vi "non recursive akhil2.vi"() -> ()   [LabVIEW 2014]
uses:
  <vilib>/LabVIEW Targets/FPGA/cRIO/shared/nicrio_ModuleControls/nicrio_cRIO-9467_Altitude.ctl
  <vilib>/LabVIEW Targets/FPGA/cRIO/shared/nicrio_ModuleControls/nicrio_cRIO-9467_Longitude.ctl
  <vilib>/LabVIEW Targets/FPGA/cRIO/shared/nicrio_ModuleControls/nicrio_cRIO-9467_Latitude.ctl
  <vilib>/LabVIEW Targets/FPGA/cRIO/shared/nicrio_ModuleControls/nicrio_cRIO-9225_DataRatesRing.ctl
  <vilib>/LabVIEW Targets/FPGA/cRIO/shared/nicrio_ModuleControls/nicrio_cRIO-9227_DataRatesRing.ctl
  <vilib>/Platform/TimedLoop/XDataNode/timing_clust.ctl
  <vilib>/Platform/TimedLoop/XDataNode/nitl_modes.ctl
  <vilib>/Platform/TimedLoop/XDataNode/wakeup.ctl
  <vilib>/rvi/FXPMathLib/FxpSinAndCos/subVIs/nifxpmath_SinAndCos_SimConfig.ctl
  <vilib>/rvi/FXPMathLib/FxpRectToPolar/subVIs/nifxpmath_RectToPolar_SimConfig.ctl
  <vilib>/rvi/Emulation/niFpgaGetClockAttributes.vi
  <vilib>/rvi/Emulation/niFpgaSctlEmulationGetInTimedLoop.vi
  <vilib>/rvi/Emulation/niFpgaEmulationReportErrorSimple.vi
  <vilib>/rvi/eio/common/nirviEmuTemplateMethod_errors.vi
  <vilib>/rvi/eio/common/nirviEmuTemplatePropertyGet_noerrors.vi
  <vilib>/rvi/Emulation/niFpgaCriticalErrorInLSC.vi
  <vilib>/rvi/Memory/Memory_Emulation/nirvimemoryFastEmulation.vi
  <vilib>/rvi/Memory/Memory_Emulation/nirvimemoryEmulation.vi
  <vilib>/rvi/Emulation/niFpgaEmulationIsFPGAContextNoSignature.vi
  <vilib>/rvi/DataTransferAndStorage/Container/Common/niFpgaContainerGetUniqueNameForEmu.vi
  <vilib>/rvi/Emulation/niFpgaProcessEmulError.vi
  <vilib>/rvi/errors/nirviReportUnexpectedCaseInternalError (U32).vi
  <vilib>/rvi/FXPMathLib/FxpSinAndCos/simVIs/DllFxpSinAndCosTemp_sub.vi
  <vilib>/rvi/FXPMathLib/FxpRectToPolar/simVIs/DllFxpRectToPolarTemp_sub.vi
  <vilib>/rvi/DataTransferAndStorage/Container/Common/niFpgaContainerSetEmuInfo.vi
  <vilib>/rvi/eio/common/nirviEmuReportErrorAndStop.vi
  <vilib>/rvi/eio/common/nirviEmuTemplatePropertySet_noerrors.vi
  <vilib>/rvi/eio/common/nirviEmuTemplatePropertyGet_errors.vi
  <vilib>/eio/EIOMethodNode/EIOMethodNode.xnode
  <vilib>/eio/EIOPropertyNode/EIOPropertyNode.xnode
  <vilib>/eio/EIONode/EIONode.xnode
  <vilib>/Platform/TimedLoop/XDataNode/XDataNode.xnode
  <vilib>/rvi/DataTransferAndStorage/Container/XNode/niFpgaContainer.xnode
  <vilib>/rvi/FXPMathLib/FxpMul/XNode/nifxpmath_Multiplier.xnode
  <vilib>/rvi/FXPMathLib/FxpSinAndCos/XNode/nifxpmath_SinAndCos.xnode
  <vilib>/rvi/FXPMathLib/FxpAdd/XNode/nifxpmath_Add.xnode
  <vilib>/rvi/FXPMathLib/FxpRectToPolar/XNode/nifxpmath_RectToPolar.xnode
  <vilib>/rvi/LocalResourceManager/LocalResourceManager.xnode
  <vilib>/rvi/FXPMathLib/sim/FxpSim.dll
  <vilib>/Platform/TimedLoop/XDataNode/XDNodeRunTimeDep.lvlib
  <vilib>/rvi/eio/common/nirviEmuTemplatePropertySet_errors.vi
  fpga timekeeper/FPGA Timekeeper.lvlib
panel:
  out "Firmware Version":u32 format="%.0x"
  out "Vendor ID":u16 format="%.0x"
  out "Module ID":u16 format="%.0x"
  out "Serial Number":u32 format="%.0x"
  out "FPGA Error Out":errorcluster
  in  "stop 2":bool
  out "PPS Timestamp (TAI)":u64
  out "UTC Offset":i8
  out "UTC Offset Valid":bool
  out "GPS Status":T1(ring)
  out "Antenna Status":T2(ring)
  out "Leap Second Direction":enum8{"Add", "Delete"}(ring)
  out "Leap Second Pending":bool
  out "Leap Second Occurred":bool
  out "Satellites Available":u8
  out "Self-Survey Complete":bool
  out "Latitude (°)":T3 format="%.6f"
  out "Longitude (°)":T4 format="%.6g"
  out "Altitude (m)":T5 format="%.2f"
  out "Timed Out":bool
  out "Iterations":i32
  out "FPGA Timekeeper time (ns)":u64
  out "GPS status":T1(ring)
  out "FPGA Timekeeper locked":bool
  out "offset from time reference":i32
  out "antenna status":T2(ring)
  out "satellites available":u8
  out "UTC offset":i8
  out "UTC offset valid":bool
  out "rate of chage of frequency":fxp<+/-,26,12>
  out "phase current":fxp<+/-,26,12>
  out "phase voltage":fxp<+/-,26,12>
  out "current frequency":fxp<+/-,50,19>
  out "voltage frequency":fxp<+/-,50,19>
  out "sdft magnitude":fxp<+/-,25,11>[](array[numeric])
  out "sdft phase":fxp<+/-,25,11>[](array[numeric])
  out "y phase voltage":T6(array[cluster])
  out "y phase current":T6(array[cluster])
  out "r phase current":T6(array[cluster])
  out "r phase voltage":T6(array[cluster])
  out "b phase current":T6(array[cluster])
  out "b phase voltage":T6(array[cluster])
  out "Array":T7(array[cluster])
  out "theta":fxp<+/-,22,10>[](array[numeric])
  out "r":fxp<+,60,17>[](array[numeric])
  in  "stop":bool
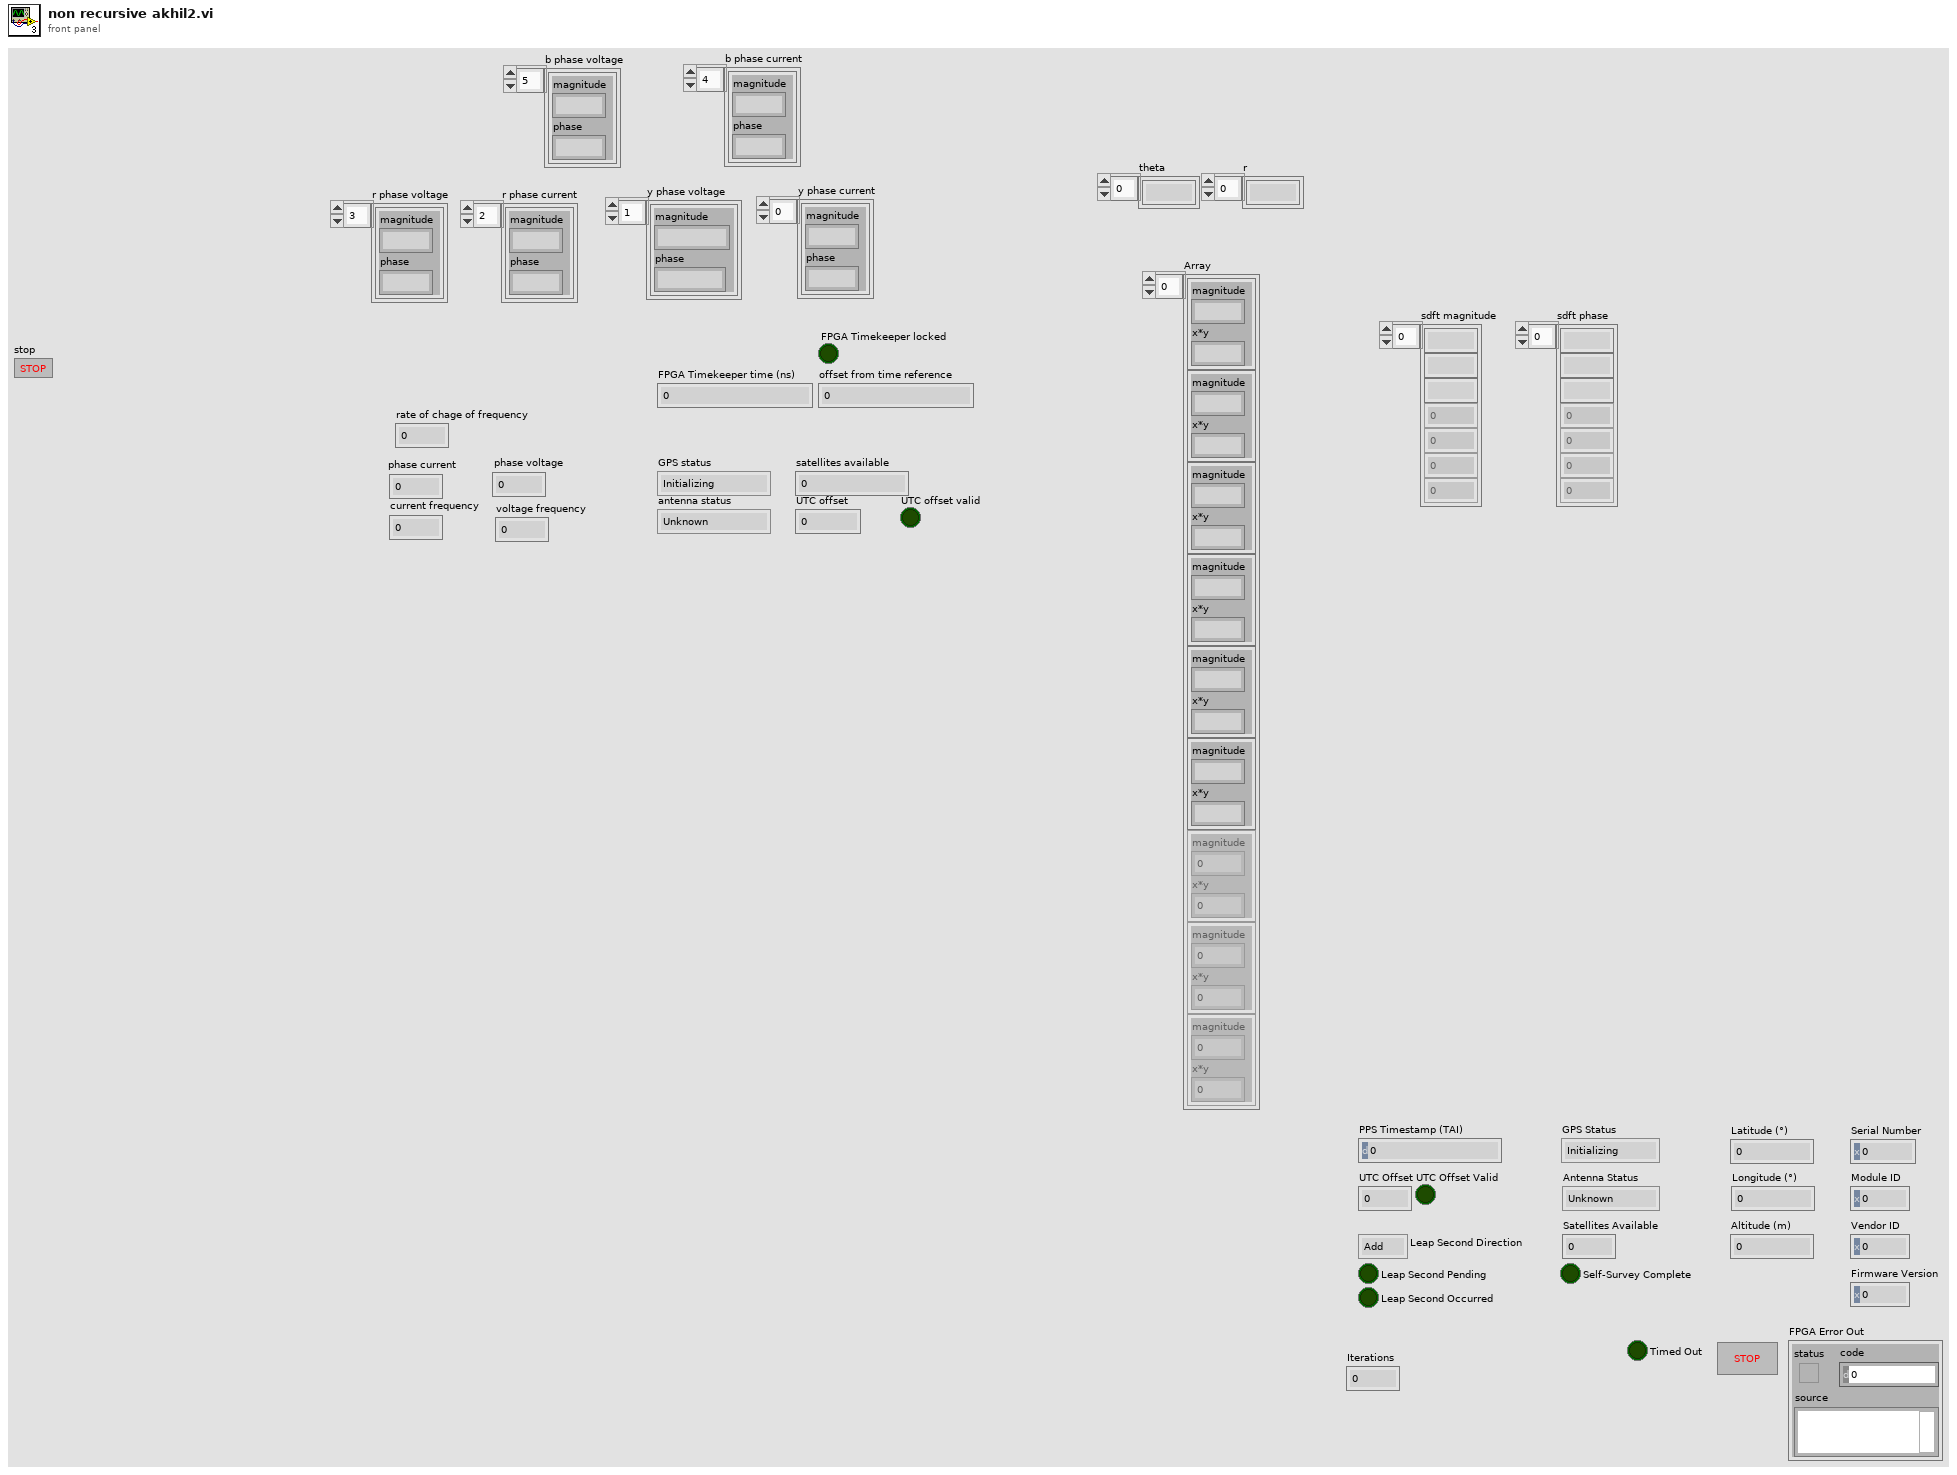
[diagram p1: front panel]
types:
  T1 = enum8{"Initializing", "Normal", "Unable to get fix"}
  T2 = enum8{"Unknown", "Normal", "Absent", "Overcurrent"}
  T3 = typedef "nicrio_cRIO-9467_Latitude.ctl" = fxp<+/-,28,8>
  T4 = typedef "nicrio_cRIO-9467_Longitude.ctl" = fxp<+/-,29,9>
  T5 = typedef "nicrio_cRIO-9467_Altitude.ctl" = fxp<+/-,24,17>
  T6 = cluster{"magnitude":fxp<+,60,17>, "phase":fxp<+/-,22,10>}[]
  T7 = cluster{"magnitude":fxp<+,60,17>, "x*y":fxp<+/-,22,10>}[]
  T8 = typedef "nicrio_cRIO-9227_DataRatesRing.ctl" = u8
  T9 = typedef "nicrio_cRIO-9225_DataRatesRing.ctl" = u8
  T10 = typedef "XDNodeRunTimeDep.lvlib/timing_clust.ctl" = cluster{"Expected End [f-1]":u64, "Actual End [f-1]":u64, "Finished Late? [f-1]":bool, "Expected End [i-1]":u64, "Actual End [i-1]":u64, "Finished Late? [i-1]":bool, "Expected Start [i]":u64, "Actual Start [i]":u64, "Expected Start [f]":u64, "Actual Start [f]":u64, "Source Name":string, "Structure Name":string, "Period":i64, "Deadline":i64, "Offset":i64, "Start":i64, "Priority":i32, "Timeout":i32, "Mode":T11, "Wakeup Reason":T12, "Error":errorcluster, "Source Type":string, "Secondary Source Type":string, "Global End Time":u64, "Global Start Time":u64, "Frame Duration":u64, "Iteration Duration":u64, "Assigned CPU":i32, "I/O Scan Engine Mode":u32}
  T11 = typedef "XDNodeRunTimeDep.lvlib/nitl_modes.ctl" = enum32{"No Change", "Process missed periods, maintain original phase", "Discard missed periods, maintain original phase", "Process missed periods, ignore original phase", "Discard missed periods, ignore original phase"}
  T12 = typedef "XDNodeRunTimeDep.lvlib/wakeup.ctl" = enum32{"Normal", "Aborted", "Asynchronous wakeup", "Timing source error", "Timed loop error", "Timeout"}
  T13 = cluster{"magnitude":fxp<+,60,17>, "x*y":fxp<+/-,22,10>}
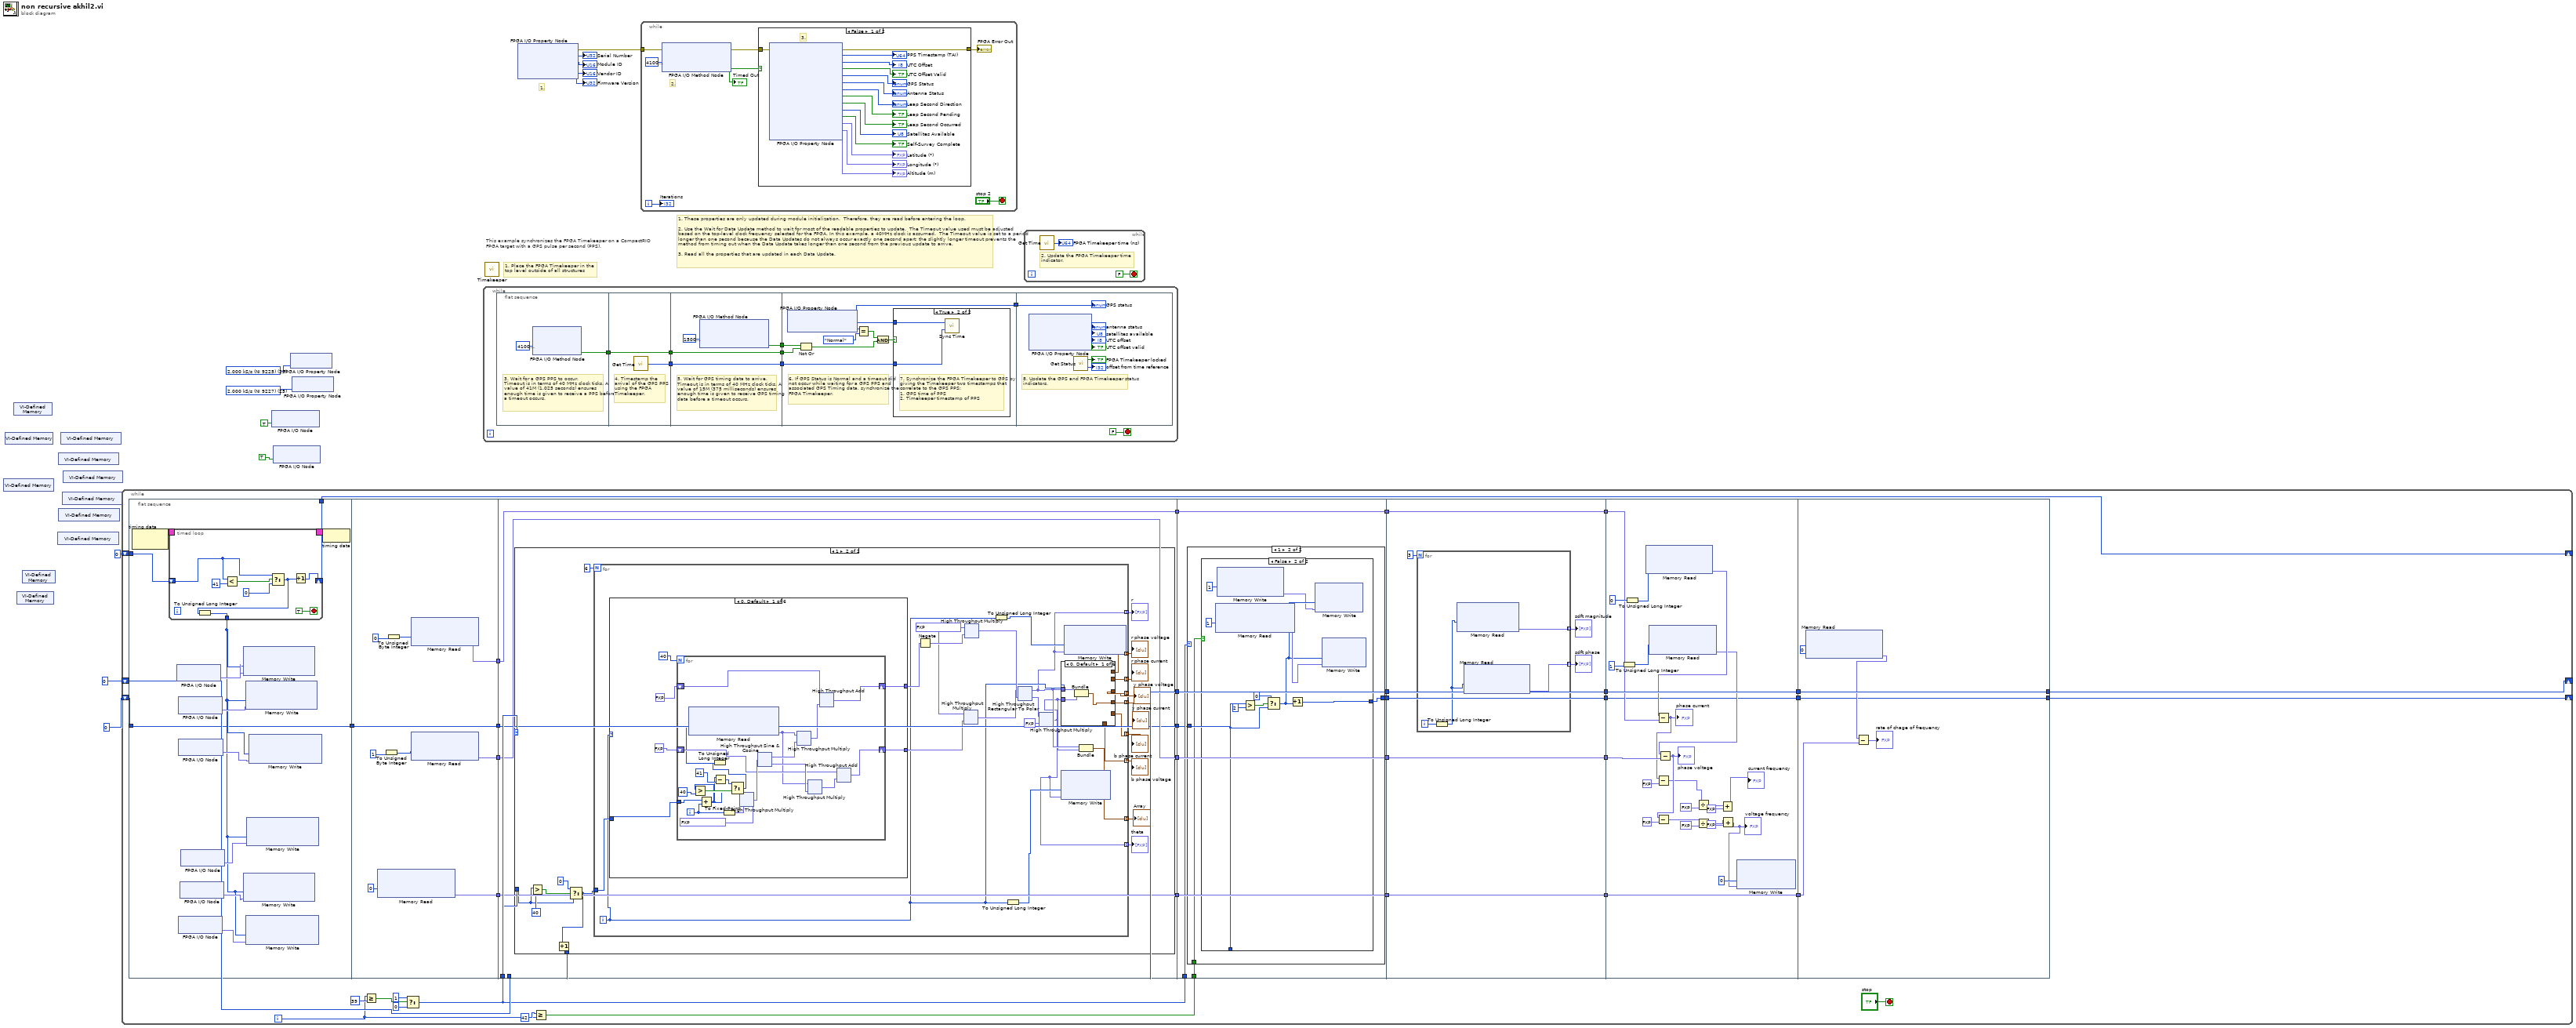
[diagram p0: block diagram]
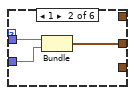
[diagram p5: hidden frame]
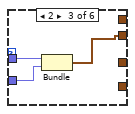
[diagram p6: hidden frame]
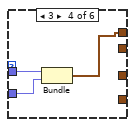
[diagram p7: hidden frame]
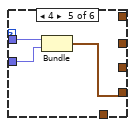
[diagram p8: hidden frame]
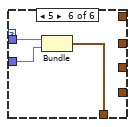
[diagram p9: hidden frame]
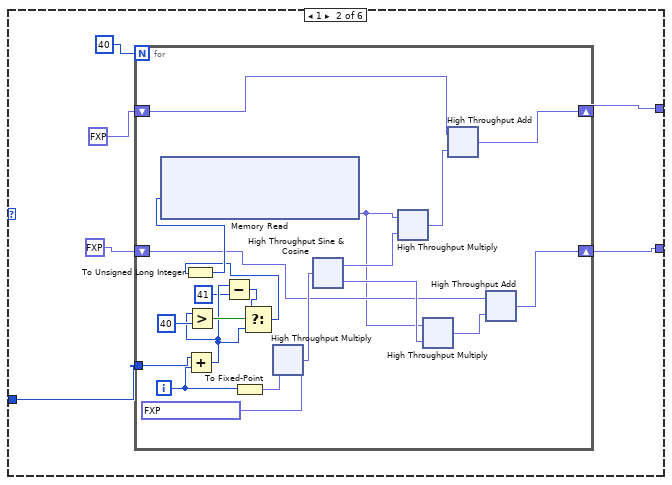
[diagram p10: hidden frame]
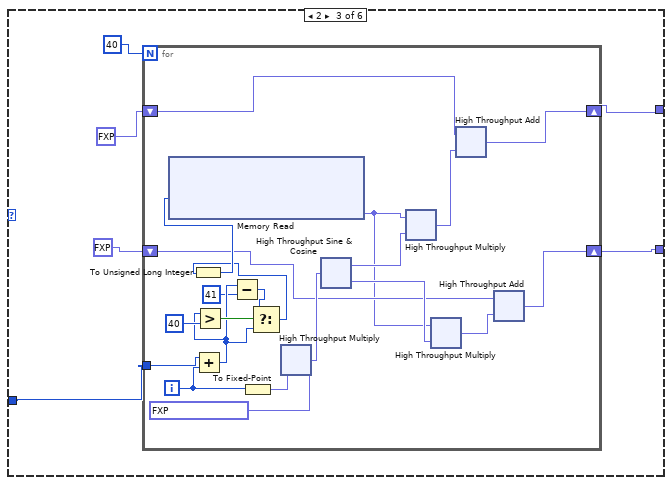
[diagram p11: hidden frame]
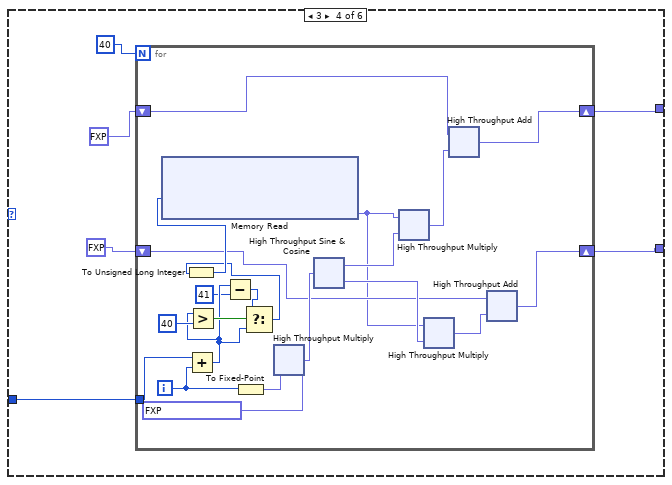
[diagram p12: hidden frame]
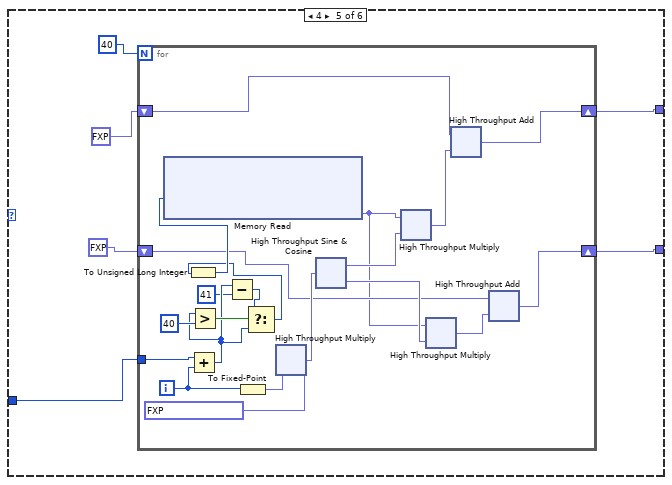
[diagram p13: hidden frame]
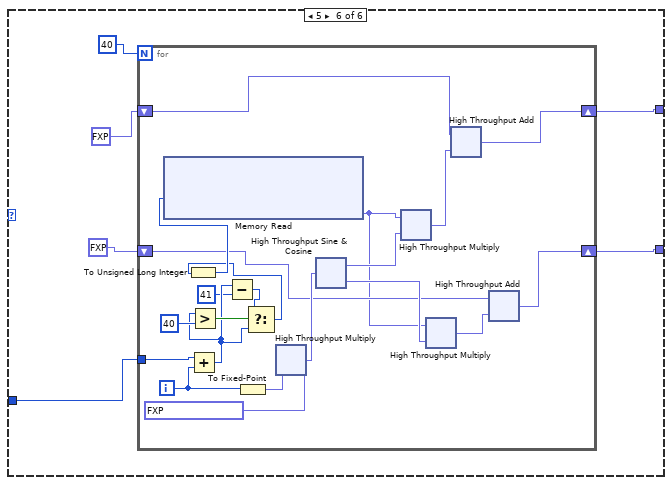
[diagram p14: hidden frame]
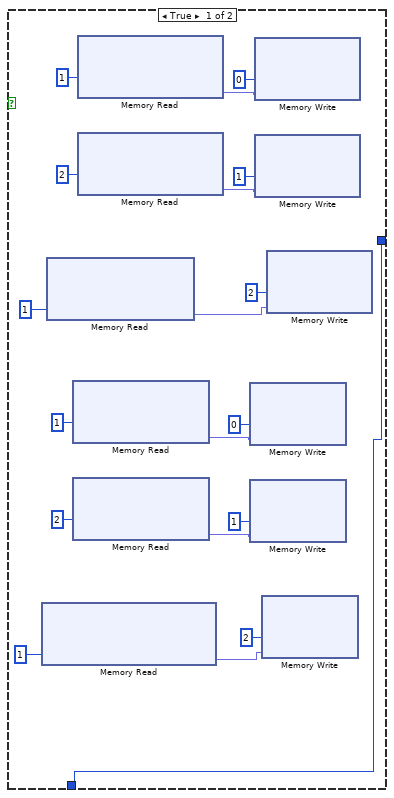
[diagram p16: hidden frame]
diagram:
  w11 = T8 25 items=["50.000 kS/s (NI 9227)"=1, "25.000 kS/s (NI 9227)"=2, "16.667 kS/s (NI 9227)"=3, "12.500 kS/s (NI 9227)"=4, "10.000 kS/s (NI 9227)"=5, "8.333 kS/s (NI 9227)"=6, "7.143 kS/s (NI 9227)"=7, "6.250 kS/s (NI 9227)"=8, "5.556 kS/s (NI 9227)"=9, "5.000 kS/s (NI 9227)"=10, "4.545 kS/s (NI 9227)"=11, "4.167 kS/s (NI 9227)"=12, "3.846 kS/s (NI 9227)"=13, "3.571 kS/s (NI 9227)"=14, "3.333 kS/s (NI 9227)"=15, "3.125 kS/s (NI 9227)"=16, "2.941 kS/s (NI 9227)"=17, "2.778 kS/s (NI 9227)"=18, "2.632 kS/s (NI 9227)"=19, "2.500 kS/s (NI 9227)"=20, "2.381 kS/s (NI 9227)"=21, "2.273 kS/s (NI 9227)"=22, "2.174 kS/s (NI 9227)"=23, "2.083 kS/s (NI 9227)"=24, "2.000 kS/s (NI 9227)"=25, "1.923 kS/s (NI 9227)"=26, "1.852 kS/s (NI 9227)"=27, "1.786 kS/s (NI 9227)"=28, "1.724 kS/s (NI 9227)"=29, "1.667 kS/s (NI 9227)"=30, "1.613 kS/s (NI 9227)"=31] ("Data Rate")
  w8 = T9 25 items=["50.000 kS/s (NI 9225)"=1, "25.000 kS/s (NI 9225)"=2, "16.667 kS/s (NI 9225)"=3, "12.500 kS/s (NI 9225)"=4, "10.000 kS/s (NI 9225)"=5, "8.333 kS/s (NI 9225)"=6, "7.143 kS/s (NI 9225)"=7, "6.250 kS/s (NI 9225)"=8, "5.556 kS/s (NI 9225)"=9, "5.000 kS/s (NI 9225)"=10, "4.545 kS/s (NI 9225)"=11, "4.167 kS/s (NI 9225)"=12, "3.846 kS/s (NI 9225)"=13, "3.571 kS/s (NI 9225)"=14, "3.333 kS/s (NI 9225)"=15, "3.125 kS/s (NI 9225)"=16, "2.941 kS/s (NI 9225)"=17, "2.778 kS/s (NI 9225)"=18, "2.632 kS/s (NI 9225)"=19, "2.500 kS/s (NI 9225)"=20, "2.381 kS/s (NI 9225)"=21, "2.273 kS/s (NI 9225)"=22, "2.174 kS/s (NI 9225)"=23, "2.083 kS/s (NI 9225)"=24, "2.000 kS/s (NI 9225)"=25, "1.923 kS/s (NI 9225)"=26, "1.852 kS/s (NI 9225)"=27, "1.786 kS/s (NI 9225)"=28, "1.724 kS/s (NI 9225)"=29, "1.667 kS/s (NI 9225)"=30, "1.613 kS/s (NI 9225)"=31] ("Data Rate")
  # "1."
  # "1. These properties are only updated during module initialization.  Therefore, they are read before entering the loop.\n\n2. Use the Wait for Data Update method to wait for most of the readable properties to update.  The Timeout value used must be adjusted based on the top-level clock frequency selected for the FPGA. In this example, a 40MHz clock is assumed.  The Timeout value is set to a period longer than one second because the Data Updates do not always occur exactly one second apart; the slightly longer timeout prevents the method from timing out when the Data Update takes longer than one second from the previous update to arrive. \n\n3. Read all the properties that are updated in each Data Update."
  # "This example synchronizes the FPGA Timekeeper on a CompactRIO FPGA target with a GPS pulse per second (PPS)."
  # "1. Place the FPGA Timekeeper in the\ntop level outside of all structures"
  n1 = xnode "VI-Defined Memory"() -> ()  [unwired: 1 out]
  n2 = xnode "VI-Defined Memory"() -> ()  [unwired: 1 out]
  n3 = xnode "VI-Defined Memory"() -> ()  [unwired: 1 out]
  n4 = xnode "VI-Defined Memory"() -> ()  [unwired: 1 out]
  n5 = xnode "VI-Defined Memory"() -> ()  [unwired: 1 out]
  n6 = xnode "VI-Defined Memory"() -> ()  [unwired: 1 out]
  n7 = xnode "VI-Defined Memory"() -> ()  [unwired: 1 out]
  n8 = xnode "VI-Defined Memory"() -> ()  [unwired: 1 out]
  n9 = xnode "VI-Defined Memory"() -> ()  [unwired: 1 out]
  n10 = xnode "VI-Defined Memory"() -> ()  [unwired: 1 out]
  n11 = xnode "VI-Defined Memory"() -> ()  [unwired: 1 out]
  n12 = while {
    shift-right: [w48] -> _
    shift-left: i16 0 -> [w49]
    shift-right: [w42] -> _
    shift-left: u32 0 ("t") -> [w43]
    shift-right: [w21] -> _
    shift-left: u32 0 ("t") -> [w33]
    i -> [w20]
    stop <- "stop" stop-if-true
    n13 = flat-sequence {
      tunnel: w49 -> [w61]
      tunnel: [w60] -> w48
      tunnel: [w51] -> w34
      tunnel: w33 -> [w51]
      tunnel: [w79] -> w41
      tunnel: [w78] -> w40
      tunnel: [w76] -> w37
      tunnel: [w75] -> w35
      tunnel: w34 -> [w75]
      tunnel: w36 -> [w90]
      tunnel: w43 -> [w89]
      tunnel: [w88] -> w17
      tunnel: w41 -> [w87]
      tunnel: [w87] -> w16
      tunnel: [w86] -> w15
      tunnel: w40 -> [w86]
      tunnel: [w85] -> w14
      tunnel: w37 -> [w85]
      tunnel: [w84] -> w13
      tunnel: w35 -> [w84]
      tunnel: w17 -> [w533]
      tunnel: [w533] -> w31
      tunnel: w16 -> [w532]
      tunnel: [w532] -> w29
      tunnel: w15 -> [w531]
      tunnel: [w531] -> w27
      tunnel: w14 -> [w530]
      tunnel: [w530] -> w25
      tunnel: w36 -> [w529]
      tunnel: w13 -> [w528]
      tunnel: [w527] -> w23
      tunnel: w18 -> [w526]
      tunnel: w31 -> [w574]
      tunnel: [w574] -> w30
      tunnel: w29 -> [w573]
      tunnel: [w573] -> w28
      tunnel: w27 -> [w572]
      tunnel: [w572] -> w26
      tunnel: w25 -> [w571]
      tunnel: [w571] -> w24
      tunnel: w23 -> [w570]
      tunnel: [w570] -> w22
      tunnel: w30 -> [w604]
      tunnel: w28 -> [w599]
      tunnel: w26 -> [w598]
      tunnel: [w604] -> w39
      tunnel: [w580] -> w38
      tunnel: w24 -> [w580]
      tunnel: [w579] -> w32
      tunnel: w22 -> [w579]
      tunnel: [w610] -> w42
      tunnel: w39 -> [w610]
      tunnel: w38 -> [w608]
      tunnel: [w605] -> w21
      tunnel: w32 -> [w605]
      frame #0 {
        n14 = node-c288() -> (w53:T10)  [unwired: 1 in]
        n15 = timed-loop {
          timing: w53 -> [_]
          timing-out: [_] -> w52
          tunnel: [w64] -> w54
          shift-right: [w65] -> w60
          shift-left: w61 -> [w66]
          stop <- TRUE stop-if-true
          n16 = Less?(x=w66, y=i16 41) -> (x < y?=w69:bool)
          n17 = Select(t=w66, s=w69, f=i16 0) -> (s? t:f=w67:i16)
          n18 = To Unsigned Long Integer(number=w67) -> (unsigned 32bit integer=w64:u32)
          n19 = Increment(x=w67) -> (x+1=w65:i16)
        }
        n20 = xnode "FPGA I/O Node"() -> ("Mod2/AI1"=w59:fxp<+/-,24,5>)  [unwired: 1 in, 1 out]
        n21 = xnode "FPGA I/O Node"() -> ("Mod2/AI0"=w56:fxp<+/-,24,5>)  [unwired: 1 in, 1 out]
        n22 = xnode "FPGA I/O Node"() -> ("Mod1/AI2"=w57:fxp<+/-,24,10>)  [unwired: 1 in, 1 out]
        n23 = xnode "FPGA I/O Node"() -> ("Mod2/AI2"=w55:fxp<+/-,24,5>)  [unwired: 1 in, 1 out]
        n24 = xnode "FPGA I/O Node"() -> ("Mod1/AI0"=w58:fxp<+/-,24,10>)  [unwired: 1 in, 1 out]
        n25 = xnode "FPGA I/O Node"() -> ("Mod1/AI1"=w62:fxp<+/-,24,10>)  [unwired: 1 in, 1 out]
        n26 = xnode ("Memory Write")("Address"=w54, "Data"=w59) -> ()  [unwired: 1 in, 1 out]
        n27 = xnode ("Memory Write")("Address"=w54, "Data"=w58) -> ()  [unwired: 1 in, 1 out]
        n28 = xnode ("Memory Write")("Address"=w54, "Data"=w56) -> ()  [unwired: 1 in, 1 out]
        n29 = xnode ("Memory Write")("Address"=w54, "Data"=w57) -> ()  [unwired: 1 in, 1 out]
        n30 = xnode ("Memory Write")("Address"=w54, "Data"=w62) -> ()  [unwired: 1 in, 1 out]
        n31 = xnode ("Memory Write")("Address"=w54, "Data"=w55) -> ()  [unwired: 1 in, 1 out]
        n32 = node-c288(w52) -> ()
      }
      frame #1 {
        n33 = xnode ("Memory Read")("Address"=u32 0) -> ("Data"=w76:fxp<+/-,25,11>)  [unwired: 1 in, 1 out]
        n34 = To Unsigned Byte Integer(number=i16 1) -> (unsigned 8bit integer=w80:u8)
        n35 = To Unsigned Byte Integer(number=i16 0) -> (unsigned 8bit integer=w82:u8)
        n36 = xnode ("Memory Read")("Address"=w82) -> ("Data"=w79:fxp<+/-,25,11>)  [unwired: 1 in, 1 out]
        n37 = xnode ("Memory Read")("Address"=w80) -> ("Data"=w78:fxp<+/-,25,11>)  [unwired: 1 in, 1 out]
      }
      frame #2 {
        n38 = case shown="1" w90 {
          tunnel: w89 -> [w91 w102]
          tunnel: [w91 w105] -> w88
          frame 0, Default {
          }
          frame 1 {
            n39 = Greater?(x=w102, y=u32 40) -> (0:w103:bool)
            n40 = Select(t=u32 0, s=w103, f=w102) -> (s? t:f=w100:u32)
            n41 = Increment(x=w100) -> (x+1=w105:u32)
            n42 = for {
              N: 6 -> [_]
              tunnel: [w121] -> w106 mode=indexing
              tunnel: w100 -> [w120]
              tunnel: [w116] -> w99 mode=indexing
              tunnel: [w115] -> w98 mode=indexing
              tunnel: [w114] -> w97 mode=indexing
              tunnel: [w113] -> w96 mode=indexing
              tunnel: [w112] -> w95 mode=indexing
              tunnel: [w110] -> w94 mode=indexing
              tunnel: [w108] -> w93 mode=indexing
              tunnel: [w109] -> w92 mode=indexing
              i -> [w117]
              w127 = fxp<+/-,16,1> 0.03533935546875 ("x")
              n43 = case shown="0, Default" w117 {
                tunnel: [w185 w241 w298 w355 w412 w469] -> w122
                tunnel: w120 -> [w184 w243 w300 w357 w414 w471]
                tunnel: [w186 w242 w299 w356 w413 w470] -> w119
                frame 0, Default {
                  n44 = for {
                    N: 40 ("Numeric") -> [_]
                    shift-right: [w203] -> w185
                    shift-left: fxp<+,1,1> 0.0 ("x+y") -> [w202]
                    shift-right: [w206] -> w186
                    shift-left: fxp<+,1,1> 0.0 -> [w201]
                    tunnel: w184 -> [w193]
                    i -> [w194]
                    n45 = Add(x=w193, y=w194) -> (x+y=w192:u32)
                    n46 = Greater?(x=w192, y=u32 40) -> (0:w197:bool)
                    n47 = Subtract(x=w192, y=u32 41) -> (x-y=w195:u32)
                    n48 = To Fixed-Point(number=w194) -> (fixed-point=w210:fxp<+/-,32,32>)  [unwired: 1 in]
                    n49 = Select(t=w195, s=w197, f=w192) -> (s? t:f=w191:u32)
                    n50 = To Unsigned Long Integer(number=w191) -> (unsigned 32bit integer=w190:u32)
                    n51 = xnode ("Memory Read")("Address"=w190) -> ("Data"=w199:fxp<+/-,25,11>)  [unwired: 1 in, 1 out]
                    n52 = xnode ("High Throughput Multiply")("x"=fxp<+/-,32,16> 0.04998779296875 ("number"), "y"=w210) -> ("x*y"=w209:fxp<+/-,64,48>)
                    n53 = xnode "High Throughput Sine & Cosine"("x (pi)"=w209) -> ("sin(x)"=w208:fxp<+/-,16,2>, "cos(x)"=w205:fxp<+/-,16,2>)
                    n54 = xnode ("High Throughput Multiply")("x"=w199, "y"=w208) -> ("x*y"=w207:fxp<+/-,41,13>)
                    n55 = xnode ("High Throughput Multiply")("x"=w199, "y"=w205) -> ("x*y"=w204:fxp<+/-,41,13>)
                    n56 = xnode ("High Throughput Add")("x"=w201, "y"=w207) -> ("x+y"=w206:fxp<+/-,42,14>)
                    n57 = xnode ("High Throughput Add")("x"=w202, "y"=w204) -> ("x+y"=w203:fxp<+/-,44,16>)
                  }
                }
                frame 1 {
                  n58 = for {
                    N: 40 ("Numeric") -> [_]
                    shift-right: [w259] -> w241
                    shift-left: fxp<+,1,1> 0.0 ("x+y") -> [w258]
                    shift-right: [w262] -> w242
                    shift-left: fxp<+,1,1> 0.0 -> [w257]
                    tunnel: w243 -> [w254]
                    i -> [w253]
                    n59 = Add(x=w254, y=w253) -> (x+y=w249:u32)
                    n60 = Greater?(x=w249, y=u32 40) -> (0:w251:bool)
                    n61 = Subtract(x=w249, y=u32 41) -> (x-y=w247:u32)
                    n62 = To Fixed-Point(number=w253) -> (fixed-point=w266:fxp<+/-,32,32>)  [unwired: 1 in]
                    n63 = Select(t=w247, s=w251, f=w249) -> (s? t:f=w250:u32)
                    n64 = To Unsigned Long Integer(number=w250) -> (unsigned 32bit integer=w267:u32)
                    n65 = xnode ("Memory Read")("Address"=w267) -> ("Data"=w255:fxp<+/-,25,11>)  [unwired: 1 in, 1 out]
                    n66 = xnode ("High Throughput Multiply")("x"=fxp<+/-,32,16> 0.04998779296875 ("number"), "y"=w266) -> ("x*y"=w265:fxp<+/-,64,48>)
                    n67 = xnode "High Throughput Sine & Cosine"("x (pi)"=w265) -> ("sin(x)"=w264:fxp<+/-,16,2>, "cos(x)"=w261:fxp<+/-,16,2>)
                    n68 = xnode ("High Throughput Multiply")("x"=w255, "y"=w264) -> ("x*y"=w263:fxp<+/-,41,13>)
                    n69 = xnode ("High Throughput Multiply")("x"=w255, "y"=w261) -> ("x*y"=w260:fxp<+/-,41,13>)
                    n70 = xnode ("High Throughput Add")("x"=w257, "y"=w263) -> ("x+y"=w262:fxp<+/-,42,14>)
                    n71 = xnode ("High Throughput Add")("x"=w258, "y"=w260) -> ("x+y"=w259:fxp<+/-,44,16>)
                  }
                }
                frame 2 {
                  n72 = for {
                    N: 40 ("Numeric") -> [_]
                    shift-right: [w316] -> w298
                    shift-left: fxp<+,1,1> 0.0 ("x+y") -> [w315]
                    shift-right: [w319] -> w299
                    shift-left: fxp<+,1,1> 0.0 -> [w314]
                    tunnel: w300 -> [w311]
                    i -> [w310]
                    n73 = Add(x=w311, y=w310) -> (x+y=w306:u32)
                    n74 = Greater?(x=w306, y=u32 40) -> (0:w308:bool)
                    n75 = Subtract(x=w306, y=u32 41) -> (x-y=w304:u32)
                    n76 = To Fixed-Point(number=w310) -> (fixed-point=w323:fxp<+/-,32,32>)  [unwired: 1 in]
                    n77 = Select(t=w304, s=w308, f=w306) -> (s? t:f=w307:u32)
                    n78 = To Unsigned Long Integer(number=w307) -> (unsigned 32bit integer=w324:u32)
                    n79 = xnode ("Memory Read")("Address"=w324) -> ("Data"=w312:fxp<+/-,25,11>)  [unwired: 1 in, 1 out]
                    n80 = xnode ("High Throughput Multiply")("x"=fxp<+/-,32,16> 0.04998779296875 ("number"), "y"=w323) -> ("x*y"=w322:fxp<+/-,64,48>)
                    n81 = xnode "High Throughput Sine & Cosine"("x (pi)"=w322) -> ("sin(x)"=w321:fxp<+/-,16,2>, "cos(x)"=w318:fxp<+/-,16,2>)
                    n82 = xnode ("High Throughput Multiply")("x"=w312, "y"=w321) -> ("x*y"=w320:fxp<+/-,41,13>)
                    n83 = xnode ("High Throughput Multiply")("x"=w312, "y"=w318) -> ("x*y"=w317:fxp<+/-,41,13>)
                    n84 = xnode ("High Throughput Add")("x"=w314, "y"=w320) -> ("x+y"=w319:fxp<+/-,42,14>)
                    n85 = xnode ("High Throughput Add")("x"=w315, "y"=w317) -> ("x+y"=w316:fxp<+/-,44,16>)
                  }
                }
                frame 3 {
                  n86 = for {
                    N: 40 ("Numeric") -> [_]
                    shift-right: [w373] -> w355
                    shift-left: fxp<+,1,1> 0.0 ("x+y") -> [w372]
                    shift-right: [w376] -> w356
                    shift-left: fxp<+,1,1> 0.0 -> [w371]
                    tunnel: w357 -> [w361]
                    i -> [w368]
                    n87 = Add(x=w361, y=w368) -> (x+y=w364:u32)
                    n88 = Greater?(x=w364, y=u32 40) -> (0:w366:bool)
                    n89 = Subtract(x=w364, y=u32 41) -> (x-y=w362:u32)
                    n90 = To Fixed-Point(number=w368) -> (fixed-point=w380:fxp<+/-,32,32>)  [unwired: 1 in]
                    n91 = Select(t=w362, s=w366, f=w364) -> (s? t:f=w365:u32)
                    n92 = To Unsigned Long Integer(number=w365) -> (unsigned 32bit integer=w381:u32)
                    n93 = xnode ("Memory Read")("Address"=w381) -> ("Data"=w369:fxp<+/-,25,11>)  [unwired: 1 in, 1 out]
                    n94 = xnode ("High Throughput Multiply")("x"=fxp<+/-,32,16> 0.04998779296875 ("number"), "y"=w380) -> ("x*y"=w379:fxp<+/-,64,48>)
                    n95 = xnode "High Throughput Sine & Cosine"("x (pi)"=w379) -> ("sin(x)"=w378:fxp<+/-,16,2>, "cos(x)"=w375:fxp<+/-,16,2>)
                    n96 = xnode ("High Throughput Multiply")("x"=w369, "y"=w378) -> ("x*y"=w377:fxp<+/-,41,13>)
                    n97 = xnode ("High Throughput Multiply")("x"=w369, "y"=w375) -> ("x*y"=w374:fxp<+/-,41,13>)
                    n98 = xnode ("High Throughput Add")("x"=w371, "y"=w377) -> ("x+y"=w376:fxp<+/-,42,14>)
                    n99 = xnode ("High Throughput Add")("x"=w372, "y"=w374) -> ("x+y"=w373:fxp<+/-,44,16>)
                  }
                }
                frame 4 {
                  n100 = for {
                    N: 40 ("Numeric") -> [_]
                    shift-right: [w430] -> w412
                    shift-left: fxp<+,1,1> 0.0 ("x+y") -> [w429]
                    shift-right: [w433] -> w413
                    shift-left: fxp<+,1,1> 0.0 -> [w428]
                    tunnel: w414 -> [w418]
                    i -> [w425]
                    n101 = Add(x=w418, y=w425) -> (x+y=w421:u32)
                    n102 = Greater?(x=w421, y=u32 40) -> (0:w423:bool)
                    n103 = Subtract(x=w421, y=u32 41) -> (x-y=w419:u32)
                    n104 = To Fixed-Point(number=w425) -> (fixed-point=w437:fxp<+/-,32,32>)  [unwired: 1 in]
                    n105 = Select(t=w419, s=w423, f=w421) -> (s? t:f=w422:u32)
                    n106 = To Unsigned Long Integer(number=w422) -> (unsigned 32bit integer=w438:u32)
                    n107 = xnode ("Memory Read")("Address"=w438) -> ("Data"=w426:fxp<+/-,25,11>)  [unwired: 1 in, 1 out]
                    n108 = xnode ("High Throughput Multiply")("x"=fxp<+/-,32,16> 0.04998779296875 ("number"), "y"=w437) -> ("x*y"=w436:fxp<+/-,64,48>)
                    n109 = xnode "High Throughput Sine & Cosine"("x (pi)"=w436) -> ("sin(x)"=w435:fxp<+/-,16,2>, "cos(x)"=w432:fxp<+/-,16,2>)
                    n110 = xnode ("High Throughput Multiply")("x"=w426, "y"=w435) -> ("x*y"=w434:fxp<+/-,41,13>)
                    n111 = xnode ("High Throughput Multiply")("x"=w426, "y"=w432) -> ("x*y"=w431:fxp<+/-,41,13>)
                    n112 = xnode ("High Throughput Add")("x"=w428, "y"=w434) -> ("x+y"=w433:fxp<+/-,42,14>)
                    n113 = xnode ("High Throughput Add")("x"=w429, "y"=w431) -> ("x+y"=w430:fxp<+/-,44,16>)
                  }
                }
                frame 5 {
                  n114 = for {
                    N: 40 ("Numeric") -> [_]
                    shift-right: [w487] -> w469
                    shift-left: fxp<+,1,1> 0.0 ("x+y") -> [w486]
                    shift-right: [w490] -> w470
                    shift-left: fxp<+,1,1> 0.0 -> [w485]
                    tunnel: w471 -> [w475]
                    i -> [w482]
                    n115 = Add(x=w475, y=w482) -> (x+y=w478:u32)
                    n116 = Greater?(x=w478, y=u32 40) -> (0:w480:bool)
                    n117 = Subtract(x=w478, y=u32 41) -> (x-y=w476:u32)
                    n118 = To Fixed-Point(number=w482) -> (fixed-point=w494:fxp<+/-,32,32>)  [unwired: 1 in]
                    n119 = Select(t=w476, s=w480, f=w478) -> (s? t:f=w479:u32)
                    n120 = To Unsigned Long Integer(number=w479) -> (unsigned 32bit integer=w495:u32)
                    n121 = xnode ("Memory Read")("Address"=w495) -> ("Data"=w483:fxp<+/-,25,11>)  [unwired: 1 in, 1 out]
                    n122 = xnode ("High Throughput Multiply")("x"=fxp<+/-,32,16> 0.04998779296875 ("number"), "y"=w494) -> ("x*y"=w493:fxp<+/-,64,48>)
                    n123 = xnode "High Throughput Sine & Cosine"("x (pi)"=w493) -> ("sin(x)"=w492:fxp<+/-,16,2>, "cos(x)"=w489:fxp<+/-,16,2>)
                    n124 = xnode ("High Throughput Multiply")("x"=w483, "y"=w492) -> ("x*y"=w491:fxp<+/-,41,13>)
                    n125 = xnode ("High Throughput Multiply")("x"=w483, "y"=w489) -> ("x*y"=w488:fxp<+/-,41,13>)
                    n126 = xnode ("High Throughput Add")("x"=w485, "y"=w491) -> ("x+y"=w490:fxp<+/-,42,14>)
                    n127 = xnode ("High Throughput Add")("x"=w486, "y"=w488) -> ("x+y"=w487:fxp<+/-,44,16>)
                  }
                }
              }
              n128 = Negate(x=w119) -> (-x=w128:fxp<+/-,43,15>)
              n129 = xnode ("High Throughput Multiply")("x"=w127, "y"=w122) -> ("x*y"=w123:fxp<+/-,60,17>)
              n130 = xnode ("High Throughput Multiply")("x"=w127, "y"=w128) -> ("x*y"=w124:fxp<+/-,59,16>)
              n131 = To Unsigned Long Integer(number=w117) -> (unsigned 32bit integer=w111:u32)
              n132 = To Unsigned Long Integer(number=w117) -> (unsigned 32bit integer=w118:u32)
              n133 = xnode "High Throughput Rectangular To Polar"("x"=w123, "y"=w124) -> ("magnitude"=w109:fxp<+,60,17>, "phase (pi)"=w126:fxp<+/-,16,2>)
              n134 = xnode ("High Throughput Multiply")("x"=w126, "y"=fxp<+,6,8> 180.0) -> ("x*y"=w108:fxp<+/-,22,10>)
              n135 = case shown="0, Default" w117 {
                tunnel: [_ w134 _ _ _ _] -> w121
                tunnel: w108 -> [w131 w133 w137 w140 w143 w146]
                tunnel: w109 -> [w130 w132 w136 w139 w142 w145]
                tunnel: [w129 _ _ _ _ _] -> w116
                tunnel: [_ _ w135 _ _ _] -> w115
                tunnel: [_ _ _ w138 _ _] -> w114
                tunnel: [_ _ _ _ w141 _] -> w113
                tunnel: [_ _ _ _ _ w144] -> w112
                frame 0, Default {
                  n136 = Bundle("magnitude"=w130, "x*y"=w131) -> (w129:T13)  [unwired: 1 in]
                }
                frame 1 {
                  n137 = Bundle("magnitude"=w132, "x*y"=w133) -> (w134:T13)  [unwired: 1 in]
                }
                frame 2 {
                  n138 = Bundle("magnitude"=w136, "x*y"=w137) -> (w135:T13)  [unwired: 1 in]
                }
                frame 3 {
                  n139 = Bundle("magnitude"=w139, "x*y"=w140) -> (w138:T13)  [unwired: 1 in]
                }
                frame 4 {
                  n140 = Bundle("magnitude"=w142, "x*y"=w143) -> (w141:T13)  [unwired: 1 in]
                }
                frame 5 {
                  n141 = Bundle("magnitude"=w145, "x*y"=w146) -> (w144:T13)  [unwired: 1 in]
                }
              }
              n142 = xnode ("Memory Write")("Address"=w118, "Data"=w108) -> ()  [unwired: 1 in, 1 out]
              n143 = xnode ("Memory Write")("Address"=w111, "Data"=w109) -> ()  [unwired: 1 in, 1 out]
              n144 = Bundle("magnitude"=w109, "x*y"=w108) -> (w110:T13)  [unwired: 1 in]
            }
            "y phase voltage" <- w106
            "y phase current" <- w99
            "r phase current" <- w98
            "r phase voltage" <- w97
            "b phase current" <- w96
            "b phase voltage" <- w95
            "Array" <- w94
            "theta" <- w93
            "r" <- w92
          }
        }
      }
      frame #3 {
        n145 = case shown="1" w529 {
          tunnel: w528 -> [w534 w536]
          tunnel: [w534 w537] -> w527
          tunnel: w526 -> [_ w535]
          frame 0, Default {
          }
          frame 1 {
            n146 = case shown="False" w535 {
              tunnel: [w556 w564] -> w537
              tunnel: w536 -> [w556 w561]
              frame True {
                n147 = xnode ("Memory Read")("Address"=u32 1) -> ("Data"=w538:fxp<+/-,25,11>)  [unwired: 1 in, 1 out]
                n148 = xnode ("Memory Read")("Address"=u32 1) -> ("Data"=w547:fxp<+/-,25,11>)  [unwired: 1 in, 1 out]
                n149 = xnode ("Memory Read")("Address"=u32 1) -> ("Data"=w545:fxp<+/-,25,11>)  [unwired: 1 in, 1 out]
                n150 = xnode ("Memory Read")("Address"=u32 2) -> ("Data"=w542:fxp<+/-,25,11>)  [unwired: 1 in, 1 out]
                n151 = xnode ("Memory Read")("Address"=u32 1) -> ("Data"=w554:fxp<+/-,25,11>)  [unwired: 1 in, 1 out]
                n152 = xnode ("Memory Read")("Address"=u32 2) -> ("Data"=w551:fxp<+/-,25,11>)  [unwired: 1 in, 1 out]
                n153 = xnode ("Memory Write")("Address"=u32 0, "Data"=w545) -> ()  [unwired: 1 in, 1 out]
                n154 = xnode ("Memory Write")("Address"=u32 1, "Data"=w542) -> ()  [unwired: 1 in, 1 out]
                n155 = xnode ("Memory Write")("Address"=u32 0, "Data"=w554) -> ()  [unwired: 1 in, 1 out]
                n156 = xnode ("Memory Write")("Address"=u32 1, "Data"=w551) -> ()  [unwired: 1 in, 1 out]
                n157 = xnode ("Memory Write")("Address"=u32 2, "Data"=w538) -> ()  [unwired: 1 in, 1 out]
                n158 = xnode ("Memory Write")("Address"=u32 2, "Data"=w547) -> ()  [unwired: 1 in, 1 out]
              }
              frame False {
                n159 = xnode ("Memory Read")("Address"=u32 1) -> ("Data"=w565:fxp<+/-,25,11>)  [unwired: 1 in, 1 out]
                n160 = xnode ("Memory Write")("Address"=u32 1) -> ("Data"=w557:fxp<+/-,25,11>)  [unwired: 1 in, 1 out]
                n161 = Greater?(x=w561, y=u32 2) -> (0:w562:bool)
                n162 = Select(t=u32 0, s=w562, f=w561) -> (s? t:f=w558:u32)
                n163 = Increment(x=w558) -> (x+1=w564:u32)
                n164 = xnode ("Memory Write")("Address"=w558, "Data"=w557) -> ()  [unwired: 1 in, 1 out]
                n165 = xnode ("Memory Write")("Address"=w558, "Data"=w565) -> ()  [unwired: 1 in, 1 out]
              }
            }
          }
        }
      }
      frame #4 {
        n166 = for {
          N: 3 -> [_]
          tunnel: [w577] -> w568 mode=indexing
          tunnel: [w575] -> w567 mode=indexing
          i -> [w578]
          n167 = To Unsigned Long Integer(number=w578) -> (unsigned 32bit integer=w576:u32)
          n168 = xnode ("Memory Read")("Address"=w576) -> ("Data"=w577:fxp<+/-,25,11>)  [unwired: 1 in, 1 out]
          n169 = xnode ("Memory Read")("Address"=w576) -> ("Data"=w575:fxp<+/-,25,11>)  [unwired: 1 in, 1 out]
        }
        "sdft magnitude" <- w568
        "sdft phase" <- w567
      }
      frame #5 {
        n170 = To Unsigned Long Integer(number=i16 1) -> (unsigned 32bit integer=w600:u32)
        n171 = To Unsigned Long Integer(number=i16 0) -> (unsigned 32bit integer=w602:u32)
        n172 = xnode ("Memory Read")("Address"=w602) -> ("Data"=w597:fxp<+/-,25,11>)  [unwired: 1 in, 1 out]
        n173 = xnode ("Memory Read")("Address"=w600) -> ("Data"=w596:fxp<+/-,25,11>)  [unwired: 1 in, 1 out]
        n174 = Subtract(x=w597, y=w599) -> (x-y=w588:fxp<+/-,26,12>)
        "phase current" <- w588
        n175 = Subtract(x=w588, y=fxp<+/-,17,17> 9.0) -> (x-y=w584:fxp<+/-,32,18>)
        n176 = Subtract(x=w596, y=w598) -> (x-y=w586:fxp<+/-,26,12>)
        "phase voltage" <- w586
        n177 = Subtract(x=w586, y=fxp<+/-,17,17> 9.0) -> (x-y=w583:fxp<+/-,32,18>)
        n178 = Divide(x=w584, y=fxp<+/-,17,17> 360.0) -> (x/y=w593:fxp<+/-,49,18>)
        n179 = Divide(x=w583, y=fxp<+/-,17,17> 360.0) -> (x/y=w591:fxp<+/-,49,18>)
        n180 = Add(x=w593, y=fxp<+/-,34,17> 50.0) -> (x+y=→"current frequency":fxp<+/-,50,19>)
        n181 = Add(x=w591, y=fxp<+/-,34,17> 50.0) -> (x+y=w581:fxp<+/-,50,19>)
        "voltage frequency" <- w581
        n182 = xnode ("Memory Write")("Address"=u32 0, "Data"=w581) -> ()  [unwired: 1 in, 1 out]
      }
      frame #6 {
        n183 = xnode ("Memory Read")("Address"=u32 0) -> ("Data"=w607:fxp<+/-,25,11>)  [unwired: 1 in, 1 out]
        n184 = Subtract(x=w607, y=w608) -> (x-y=→"rate of chage of frequency":fxp<+/-,26,12>)
      }
    }
    n185 = Greater Or Equal?(x=w20, y=39) -> (x >= y?=w46:bool)
    n186 = Select(t=u32 1, s=w46, f=u32 0) -> (s? t:f=w36:u32)
    n187 = Greater Or Equal?(x=w20, y=42) -> (x >= y?=w18:bool)
  }
  n188 = xnode "FPGA I/O Node"("Mod1/Start"=TRUE) -> ()  [unwired: 1 in, 1 out]
  n189 = xnode "FPGA I/O Node"("Mod2/Start"=TRUE) -> ()  [unwired: 1 in, 1 out]
  n190 = xnode "FPGA I/O Property Node"("Data Rate"=w8) -> ()  [unwired: 1 in, 1 out]
  n191 = xnode "FPGA I/O Property Node"("Data Rate"=w11) -> ()  [unwired: 1 in, 1 out]
  n192 = while {
    stop <- FALSE stop-if-true
    n193 = flat-sequence {
      tunnel: [w619] -> w617
      tunnel: w617 -> [w622]
      tunnel: [w622] -> w616
      tunnel: [w621] -> w614
      tunnel: [w625] -> w618
      tunnel: w616 -> [w624]
      tunnel: [w624] -> w615
      tunnel: w614 -> [w623]
      tunnel: [w623] -> w613
      tunnel: w618 -> [w634]
      tunnel: w615 -> [w633]
      tunnel: w613 -> [w628]
      tunnel: [w627] -> w612
      tunnel: w612 -> [w644]
      frame #0 {
        # "3. Wait for a GPS PPS to occur.\nTimeout is in terms of 40 MHz clock ticks. A value of 41M (1.025 seconds) ensures enough time is given to receive a PPS before a timeout occurs."
        n194 = xnode "FPGA I/O Method Node"("Timeout"=41000000) -> ("Timed Out"=w619:bool)  [unwired: 1 in, 1 out]
      }
      frame #1 {
        # "4. Timestamp the arrival of the GPS PPS using the FPGA Timekeeper."
        n195 = call "Get Time.vi"() -> ("time (ns)"=w621:u64)
      }
      frame #2 {
        # "5. Wait for GPS timing data to arrive.\nTimeout is in terms of 40 MHz clock ticks. A value of 15M (375 milliseconds) ensures enough time is given to receive GPS timing data before a timeout occurs."
        n196 = xnode "FPGA I/O Method Node"("Timeout"=15000000) -> ("Timed Out"=w625:bool)  [unwired: 1 in, 1 out]
      }
      frame #3 {
        # "6. If GPS Status is Normal and a timeout did not occur while waiting for a GPS PPS and associated GPS Timing data, synchronize the FPGA Timekeeper."
        n197 = xnode "FPGA I/O Property Node"() -> ("PPS Timestamp (TAI)"=w629:u64, "GPS Status"=w627:T1)  [unwired: 1 in, 1 out]
        n198 = Not Or(1:w633, 2:w634) -> (0:w631:bool)
        n199 = Equal?(x=w627, y=T1."Normal") -> (x = y?=w632:bool)
        n200 = And(x=w632, y=w631) -> (x .and. y?=w630:bool)
        n201 = case shown="True" w630 {
          tunnel: w629 -> [_ w637]
          tunnel: w628 -> [_ w636]
          frame False {
          }
          frame True {
            # "7. Synchronize the FPGA Timekeeper to GPS by giving the Timekeeper two timestamps that correlate to the GPS PPS:\n1. GPS time of PPS\n2. Timekeeper timestamp of PPS"
            n202 = call "Sync Time.vi"("FPGA Timekeeper time (ns)"=w636, "time reference time (ns)"=w637) -> ()
          }
        }
      }
      frame #4 {
        # "8. Update the GPS and FPGA Timekeeper status indicators."
        n203 = xnode "FPGA I/O Property Node"() -> ("Antenna Status"=→"antenna status":T2, "Satellites Available"=→"satellites available":u8, "UTC Offset"=→"UTC offset":i8, "UTC Offset Valid"=→"UTC offset valid":bool)  [unwired: 1 in, 1 out]
        n204 = call "Get Status.vi"() -> ("FPGA Timekeeper locked"=→"FPGA Timekeeper locked":bool, "offset from time reference"=→"offset from time reference":i32)
        "GPS status" <- w644
      }
    }
  }
  n205 = call "Timekeeper.vi"() -> ()  [unwired: 12 in]
  n206 = xnode "FPGA I/O Property Node"() -> ("error out"=w3:errorcluster, "Serial Number"=→"Serial Number":u32, "Module ID"=→"Module ID":u16, "Vendor ID"=→"Vendor ID":u16, "Firmware Version"=→"Firmware Version":u32)  [unwired: 2 in, 1 out]
  n207 = while {
    tunnel: w3 -> [w646]
    i -> [w645]
    stop <- "stop 2" stop-if-true
    # "2."
    n208 = xnode "FPGA I/O Method Node"("error in"=w646, "Timeout"=41000000) -> ("error out"=w651:errorcluster, "Timed Out"=w648:bool)  [unwired: 1 in, 1 out]
    "Timed Out" <- w648
    n209 = case shown="False" w648 {
      tunnel: w651 -> [w666 w667]
      tunnel: [w655 w667] -> w650
      frame False {
        # "3."
        n210 = xnode "FPGA I/O Property Node"("error in"=w666) -> ("error out"=w655:errorcluster, "PPS Timestamp (TAI)"=→"PPS Timestamp (TAI)":u64, "UTC Offset"=→"UTC Offset":i8, "UTC Offset Valid"=→"UTC Offset Valid":bool, "GPS Status"=→"GPS Status":T1, "Antenna Status"=→"Antenna Status":T2, "Leap Second Direction"=→"Leap Second Direction":enum8{"Add", "Delete"}, "Leap Second Pending"=→"Leap Second Pending":bool, "Leap Second Occurred"=→"Leap Second Occurred":bool, "Satellites Available"=→"Satellites Available":u8, "Self-Survey Complete"=→"Self-Survey Complete":bool, "Latitude (°)"=→"Latitude (°)":T3, "Longitude (°)"=→"Longitude (°)":T4, "Altitude (m)"=→"Altitude (m)":T5)  [unwired: 1 in, 1 out]
      }
      frame True {
      }
    }
    "FPGA Error Out" <- w650
    "Iterations" <- w645
  }
  n211 = while {
    stop <- FALSE stop-if-true
    # "2. Update the FPGA Timekeeper time indicator."
    n212 = call "Get Time.vi"() -> ("time (ns)"=→"FPGA Timekeeper time (ns)":u64)
  }
